vi "Initialize_Piezo_Stage_USB.vi"(1 "error in":errorcluster) -> (0 "error out":errorcluster)   [LabVIEW 2009]
panel:
  in  "USB settings":cluster{"S/N":string, "USB Search?":bool}={"S/N"="", "USB Search?"=TRUE}
  out "All conn. axes":string[](array[string])
  in  "Interface":u16(ring)=2 items=["RS232", "TCP/IP", "USB"]
  in  "System no.":i32=1 min=1 max=4 step=1
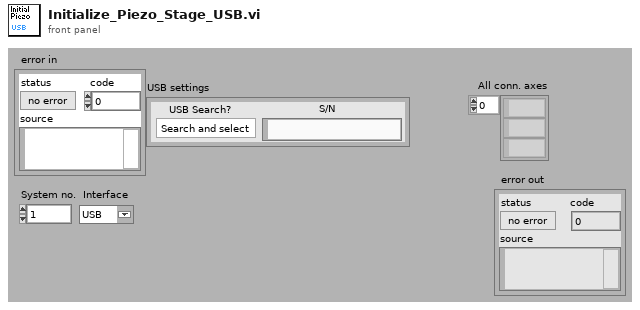
[diagram p1: front panel]
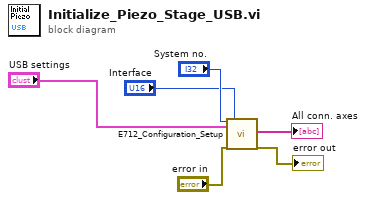
[diagram p0: block diagram]
diagram:
  n1 = call "E712_Configuration_Setup.vi"("System no."="System no.", "USB settings"="USB settings", "error in"="error in", "Interface"="Interface") -> ("All conn. axes"=→"All conn. axes":string[], "error out"=→"error out":errorcluster)  [unwired: 11 in, 3 out]
